vi "Initialize Output Channel Values.vi"(8 "error in (no error)":errorcluster, 11 "Output Process in":refnum<class "Output Process.lvclass">) -> (0 "error out":errorcluster, 3 "Output Process out":refnum<class "Output Process.lvclass">)   [LabVIEW 2019, in "TimingDRV Engine.lvlib" / "Output Process.lvclass"]
uses:
  Output Process.lvclass
  C:/Users/XEnderMD/Desktop/CD Project Tools/Source/Engine/Windows/Parent Classes/Process/Process.lvclass
  <vilib>/NI VeriStand/Custom Device API/Custom Device Channel Type.ctl
  Parent Classes/Process/Process.lvclass/Process.ctl
  Output Process.lvclass/Output Process.ctl
  Parent Classes/Process/Process.lvclass
  <vilib>/NI VeriStand/Custom Device API/Custom Device API.lvlib
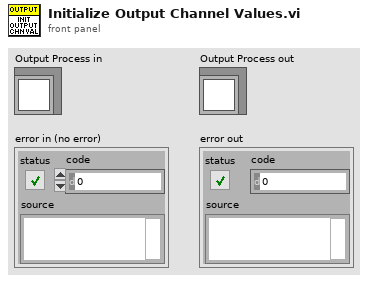
[diagram p1: front panel]
types:
  T1 = typedef "Custom Device API.lvlib/Custom Device Channel Type.ctl" = enum16{"Input", "Output"}
  T2 = typedef "Custom Device API.lvlib/Custom Device Item Ref.ctl" = u64
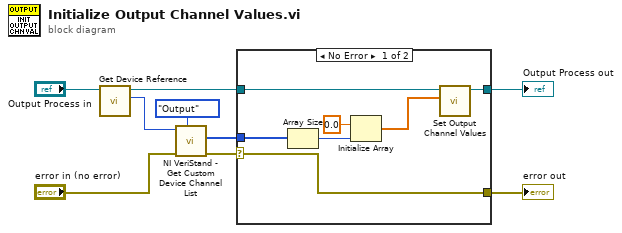
[diagram p0: block diagram]
diagram:
  n1 = call "Get Device Reference.vi"("CD_Process in"="Output Process in") -> ("Device Item Ref"=w3:T2, "CD_Process out"=w5:refnum<class "Output Process.lvclass">)  [unwired: 9 in]
  n2 = call <vilib>:"NI VeriStand - Get Custom Device Channel List.vi"("Channel Type"=Custom_Device_Channel_Type."Output", "error in (no error)"="error in (no error)", "Device Ref in"=w3) -> ("error out"=w7:errorcluster, "Specified Channel Ref List"=w4:T2[])  [unwired: 7 out]
  n3 = case shown="No Error" w7 {
    selector: w7 -> [w12 w17]
    tunnel: w4 -> [w15 _]
    tunnel: w5 -> [w14 w18]
    tunnel: [w12 w17] -> w8
    tunnel: [w11 w18] -> w9
    frame No Error {
      n4 = Array Size(array=w15) -> (size(s)=w10:i32)
      n5 = Initialize Array(0.0 ("element"), w10) -> (w13:dbl[])
      n6 = call "Set Output Channel Values.vi"("Output Channel Values"=w13, "Output Process in"=w14) -> ("Output Process out"=w11:refnum<class "Output Process.lvclass">)  [unwired: 9 in]
    }
    frame Error {
    }
  }
  "Output Process out" <- w9
  "error out" <- w8
